vi "Read flat sequences.vi"(9 "Diagram in":refnum<class "Diagram.lvclass">) -> (3 "Diagram out":refnum<class "Diagram.lvclass">, 4 "flat sequences":refnum<class "FlatSequence.lvclass">[](array[class]))   [LabVIEW 2014, in "Raspberry Pi Compatible Compiler for LabVIEW.lvlib" / "Diagram.lvclass"]
uses:
  Diagram.lvclass
  FlatSequence/FlatSequence.lvclass
  Diagram.lvclass/Diagram.ctl
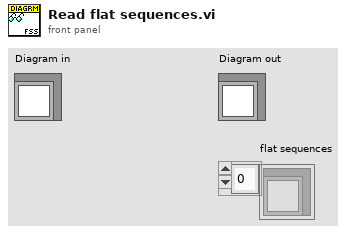
[diagram p1: front panel]
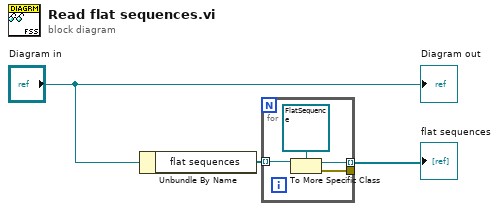
[diagram p0: block diagram]
diagram:
  n1 = Unbundle By Name("Diagram in") -> ("flat sequences"=w1:refnum<class "GObject.lvclass">[])
  n2 = for {
    tunnel: w1 -> [w7] mode=indexing
    tunnel: [w5] -> w2 mode=indexing
    tunnel: [w4] -> _
    n3 = To More Specific Class(target class=refnum<class "FlatSequence.lvclass"> refnum ("FlatSequence.lvclass"), reference=w7) -> (specific class reference=w5:refnum<class "FlatSequence.lvclass">, error out=w4:errorcluster)  [unwired: 1 in]
  }
  "flat sequences" <- w2
  "Diagram out" <- "Diagram in"
